vi "Make ISO 8601 Timestring Fractional.vi"(8 "error in (no error)":errorcluster, 10 "ISO 8601 type":T1, 11 "Time Stamp":timestamp) -> (0 "error out":errorcluster, 3 "ISO 8601 Timestring":string)   [LabVIEW 2021, in "XML Config.lvlib"]
uses:
  XML Config/XML Config.lvlib
  ISO 8601 type.ctl
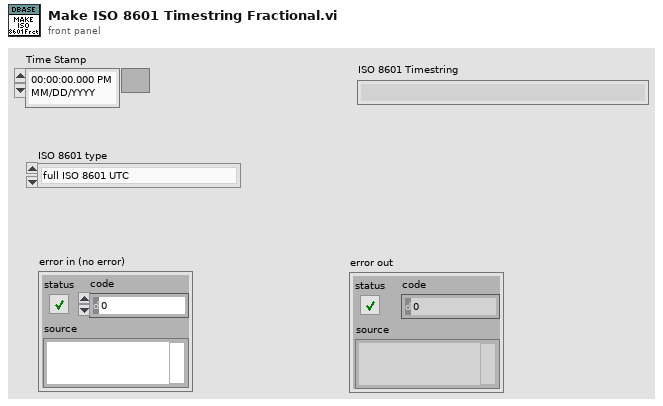
[diagram p1: front panel]
types:
  T1 = typedef "ISO 8601 type.ctl" = enum16{"full ISO 8601 UTC", "basic ISO8601 local", "Windows ISO 8601 UTC", "YYYY-MM-DD UTC", "full ISO 8601 local"}
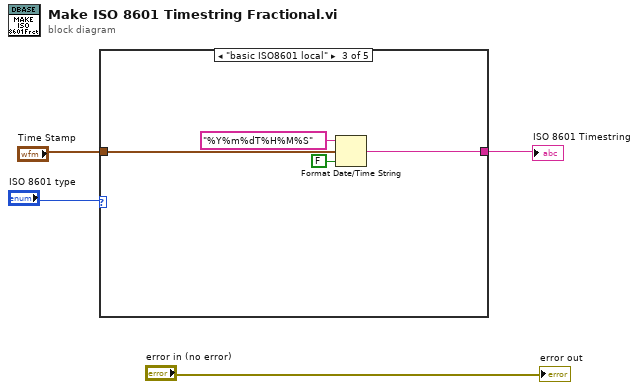
[diagram p0: block diagram]
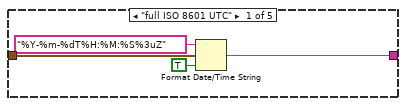
[diagram p2: hidden frame]
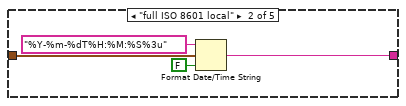
[diagram p3: hidden frame]
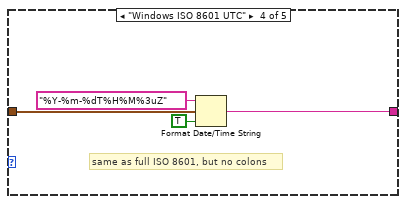
[diagram p4: hidden frame]
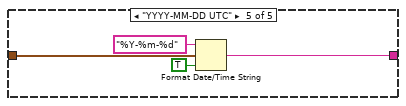
[diagram p5: hidden frame]
diagram:
  n1 = case shown="\"basic ISO8601 local\"" "ISO 8601 type" {
    tunnel: "Time Stamp" -> [w8 w12 w16 w20 w24]
    tunnel: [w6 w10 w14 w18 w22] -> w2
    frame "full ISO 8601 UTC" {
      n2 = Format Date/Time String(time format string (%c)="%Y-%m-%dT%H:%M:%S%3uZ", seconds (now)=w8, UTC format=TRUE) -> (date/time string=w6:string)
    }
    frame "full ISO 8601 local" {
      n3 = Format Date/Time String(time format string (%c)="%Y-%m-%dT%H:%M:%S%3u", seconds (now)=w12, UTC format=FALSE) -> (date/time string=w10:string)
    }
    frame "basic ISO8601 local" {
      n4 = Format Date/Time String(time format string (%c)="%Y%m%dT%H%M%S", seconds (now)=w16, UTC format=FALSE) -> (date/time string=w14:string)
    }
    frame "Windows ISO 8601 UTC" {
      # "same as full ISO 8601, but no colons"
      n5 = Format Date/Time String(time format string (%c)="%Y-%m-%dT%H%M%3uZ", seconds (now)=w20, UTC format=TRUE) -> (date/time string=w18:string)
    }
    frame "YYYY-MM-DD UTC" {
      n6 = Format Date/Time String(time format string (%c)="%Y-%m-%d", seconds (now)=w24, UTC format=TRUE) -> (date/time string=w22:string)
    }
  }
  "ISO 8601 Timestring" <- w2
  "error out" <- "error in (no error)"
